vi "Is Sub-Section of.vi"(8 "error in":errorcluster, 10 "Parent Section Name":refnum<class "Section Name.lvclass">, 11 "Section in":refnum<class "Section.lvclass">) -> (0 "error out":errorcluster, 2 "Is Sub-Section?":bool, 3 "Section out":refnum<class "Section.lvclass">)   [LabVIEW 2024, in "EDS.lvlib" / "Section.lvclass"]
uses:
  Section.lvclass
  Section Name/Section Name.lvclass
  Section.lvclass/Section.ctl
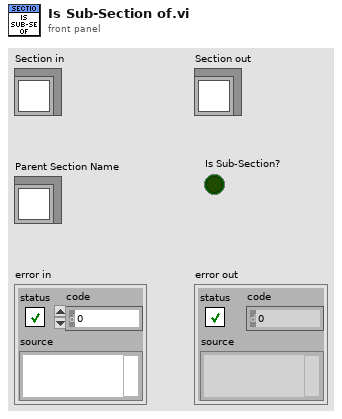
[diagram p1: front panel]
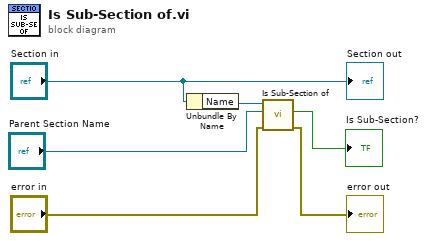
[diagram p0: block diagram]
diagram:
  n1 = Unbundle By Name("Section in") -> ("Name"=w5:refnum<class "Section Name.lvclass">)
  n2 = call "Is Sub-Section of.vi"("error in"="error in", "Parent Section Name"="Parent Section Name", "Section Name in"=w5) -> ("error out"=→"error out":errorcluster, "Is Sub-Section of?"=→"Is Sub-Section?":bool)  [unwired: 6 in, 1 out]
  "Section out" <- "Section in"
